vi "Read Msg ICS.vi"(8 "error in (no error)":errorcluster, 11 "Header content in":refnum<class "Header content.lvclass">) -> (0 "error out":errorcluster, 2 "Msg ICS":string, 3 "Header content out":refnum<class "Header content.lvclass">)   [LabVIEW 2018, in "Header content.lvclass"]
uses:
  Header content.lvclass
  Header content.lvclass/Header content.ctl
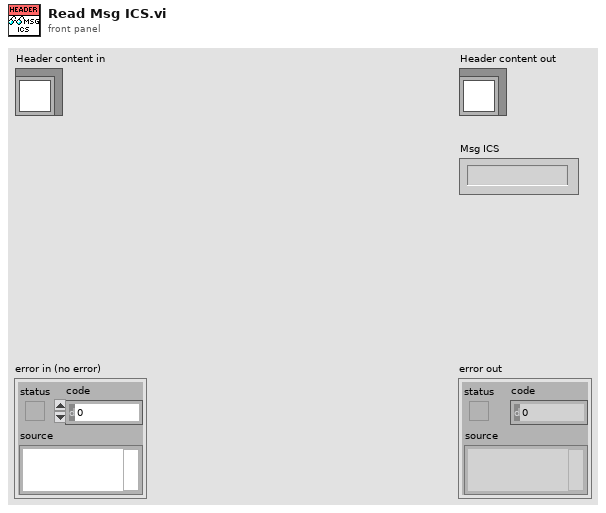
[diagram p1: front panel]
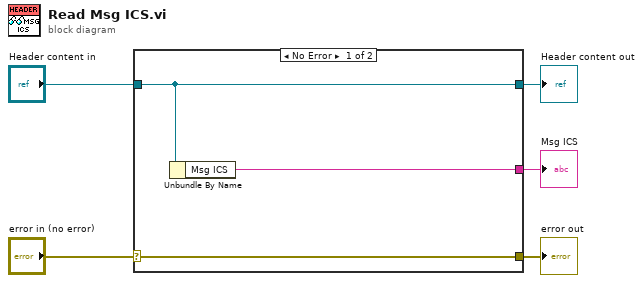
[diagram p0: block diagram]
diagram:
  n1 = case shown="No Error" "error in (no error)" {
    selector: "error in (no error)" -> [w8 w9]
    tunnel: [w8 w9] -> w4
    tunnel: [w7 w10] -> w2
    tunnel: "Header content in" -> [w7 w10]
    tunnel: [w6 _] -> w1
    frame No Error {
      n2 = Unbundle By Name(w7) -> ("Msg ICS"=w6:string)
    }
    frame Error {
    }
  }
  "error out" <- w4
  "Header content out" <- w2
  "Msg ICS" <- w1
